vi "rt_main_02_01.vi"   [LabVIEW 2015]
doc: "本模板用于队列消息处理器设计模式。\n\n事件处理循环负责按用户界面操作生成对应的消息。\n\n消息处理循环负责对事件处理循环或其他消息生成的消息进行处理。消息内容为字符串值，因此很容易将新消息添加至“消息处理”循环的“消息分支”条件结构。每个消息簇还可选择性地为消息数据提供一个变体，变体数据可以转换为消息数据所需要的任意类型。"
uses:
  globals/global_all_rt_loop_stop.vi
  globals/global_configuration_options.vi
  support_vis/message_queue/message_queue.lvlib
  <vilib>/nisyscfg/nisyscfg.lvlib
types:
  T1 = cluster{"host IP":string, "port (21)":u16, "user":string, "password":string, "remote base path":string}
  T2 = typedef "message_queue.lvlib/all_rt_message_queues.ctl" = cluster{"Queue I":refnum<queue>, "Queue II":refnum<queue>, "Queue III":refnum<queue>, "Queue IV":refnum<queue>}
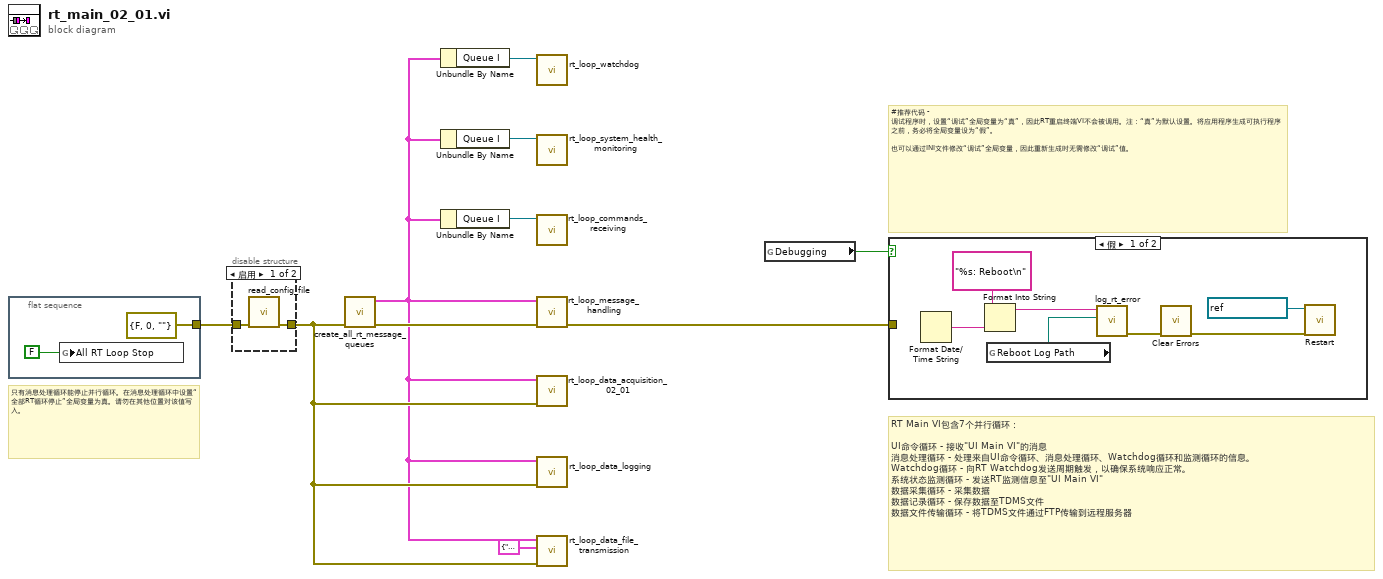
[diagram p0: block diagram]
diagram:
  # "#推荐代码 - 调试程序时，设置“调试”全局变量为“真”，因此RT重启终端VI不会被调用。注：“真”为默认设置。将应用程序生成可执行程序之前，务必将全局变量设为“假”。\n\n也可以通过INI文件修改“调试”全局变量，因此重新生成时无需修改“调试”值。"
  # "RT Main VI包含7个并行循环：\n\nUI命令循环 - 接收\"UI Main VI\"的消息\n消息处理循环 - 处理来自UI命令循环、消息处理循环、Watchdog循环和监测循环的信息。\nWatchdog循环 - 向RT Watchdog发送周期触发，以确保系统响应正常。\n系统状态监测循环 - 发送RT监测信息至\"UI Main VI\"\n数据采集循环 - 采集数据\n数据记录循环 - 保存数据至TDMS文件\n数据文件传输循环 - 将TDMS文件通过FTP传输到远程服务器"
  # "只有消息处理循环能停止并行循环。在消息处理循环中设置“全部RT循环停止”全局变量为真。请勿在其他位置对该值写入。"
  n1 = flat-sequence {
    tunnel: [errorcluster {"status"=FALSE, "code"=0, "source"=""} ("error constant")] -> w10
    frame #0 {
      n2 = global write "global_all_rt_loop_stop.vi" "All RT Loop Stop"(FALSE) -> ()
    }
  }
  n3 = disable-structure shown="启用" {
    disable-tunnel: w10 -> [w14 w15]
    disable-tunnel: [w13 w15] -> w4
    frame Enabled {
      n4 = call "read_config_file.vi"("error in (no error)"=w14) -> ("error out"=w13:errorcluster)  [unwired: 10 in]
    }
    frame Disabled {
    }
  }
  n5 = call "create_all_rt_message_queues.vi"("error in (no error)"=w4) -> ("error out"=w7:errorcluster, "Message Queues"=w2:T2)  [unwired: 9 in]
  n6 = Unbundle By Name(w2) -> ("Queue I"=w6:refnum<queue>)
  n7 = Unbundle By Name(w2) -> ("Queue I"=w3:refnum<queue>)
  n8 = Unbundle By Name(w2) -> ("Queue I"=w5:refnum<queue>)
  n9 = call "rt_loop_watchdog.vi"("Message Queue"=w6) -> ()  [unwired: 11 in]
  n10 = call "rt_loop_system_health_monitoring.vi"("Message Queue"=w3) -> ()  [unwired: 11 in]
  n11 = call "rt_loop_commands_receiving.vi"("Message Queue"=w5) -> ()  [unwired: 11 in]
  n12 = call "rt_loop_message_handling.vi"("error in (no error)"=w7, "Message Queues"=w2) -> ("error out"=w9:errorcluster)  [unwired: 9 in]
  n13 = call "rt_loop_data_acquisition_02_01.vi"("error in (no error)"=w4, "Message Queues"=w2) -> ()  [unwired: 9 in, 1 out]
  n14 = call "rt_loop_data_logging.vi"("Message Queues"=w2, "error in (no error)"=w4) -> ()  [unwired: 8 in, 1 out]
  n15 = call "rt_loop_data_file_transmission.vi"("error in (no error)"=w4, "FTP Connection Parameters"=T1 {"host IP"="192.168.16.202", "port (21)"=21, "user"="Arthur", "password"="Alin@iHome301", "remote base path"="baofu\\"}, "Message Queues"=w2) -> ()  [unwired: 8 in, 1 out]
  n16 = global read "global_configuration_options.vi" "Debugging"() -> (w8:bool)
  n17 = case shown="假" w8 {
    tunnel: w9 -> [_ _]
    frame False {
      n18 = Format Date/Time String() -> (date/time string=w20:string)  [unwired: 3 in]
      n19 = Format Into String(format string="%s: Reboot\n", w20) -> (resulting string=w19:string)  [unwired: 2 in, 1 out]
      n20 = global read "global_configuration_options.vi" "Reboot Log Path"() -> (w18:path)
      n21 = call "log_rt_error.vi"("Error Log Path"=w18, "Log Entry"=w19) -> ("error out"=w22:errorcluster)  [unwired: 9 in]
      n22 = call <vilib>:"Clear Errors.vi"("error in (no error)"=w22) -> ("error out"=w17:errorcluster)  [unwired: 5 in, 1 out]
      n23 = call <vilib>:"Restart.vi"("error in (no error)"=w17, "Session in"=refnum<k21> "localhost" ("session in")) -> ()  [unwired: 7 in, 3 out]
    }
    frame True {
    }
  }
